vi "scale kalman input.vi"(6 "t scale factor":dbl=2.5e-08, 7 "x scale factors":dbl[](array[numeric])=[0.016, 0.016, 0.00025], 10 "kalman result":T2) -> (2 "kalman result scaled":T1)   [LabVIEW 2010]
uses:
  kalman_result_unscaled.ctl
  kalman_result_scaled.ctl
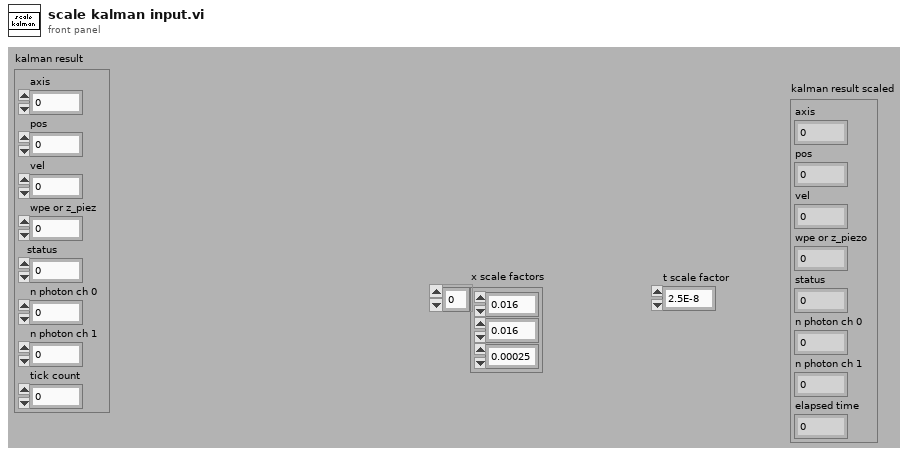
[diagram p1: front panel]
types:
  T1 = typedef "kalman_result_scaled.ctl" = cluster{"axis":u8, "pos":dbl, "vel":dbl, "wpe or z_piezo":dbl, "status":u32, "n photon ch 0":u32, "n photon ch 1":u32, "elapsed time":dbl}
  T2 = typedef "kalman_result_unscaled.ctl" = cluster{"axis":u8, "pos":i16, "vel":i16, "wpe or z_piez":i32, "status":u32, "n photon ch 0":u32, "n photon ch 1":u32, "tick count":u32}
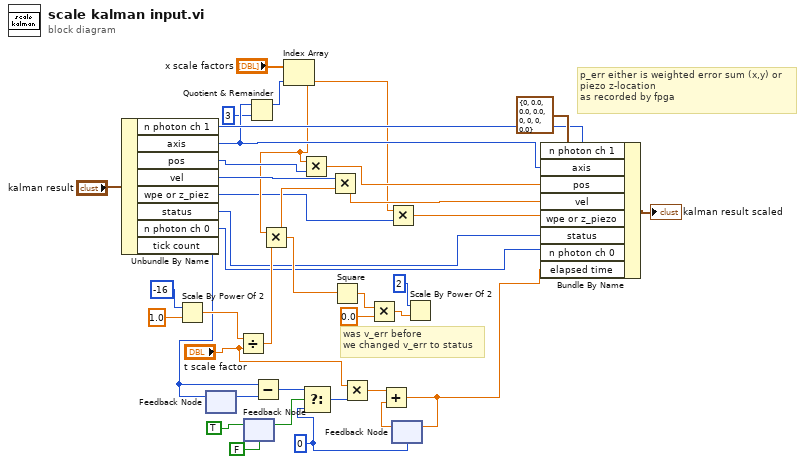
[diagram p0: block diagram]
diagram:
  w16 = 0
  # "was v_err before \nwe changed v_err to status"
  # "p_err either is weighted error sum (x,y) or\npiezo z-location \nas recorded by fpga"
  n1 = Unbundle By Name("kalman result") -> ("n photon ch 1"=w9:u32, "axis"=w6:u8, "pos"=w36:i16, "vel"=w35:i16, "wpe or z_piez"=w2:i32, "status"=w7:u32, "n photon ch 0"=w12:u32, "tick count"=w25:u32)
  n2 = Scale By Power Of 2(n=-16, x=1.0) -> (x*2^n=w32:dbl)
  n3 = feedback-in #1(w25) -> ()
  n4 = feedback #1() -> (w26:u32)  [unwired: 1 in]
  n5 = Divide(x=w32, y="t scale factor") -> (x/y=w31:dbl)
  n6 = feedback-in #2(TRUE ("s")) -> ()
  n7 = feedback #2(FALSE ("s")) -> (w21:bool)
  n8 = Quotient & Remainder(x=w6, y=u8 3) -> (x-y*floor(x/y)=w4:u8)  [unwired: 1 out]
  n9 = Subtract(x=w25, y=w26) -> (x-y=w24:u32)
  n10 = Index Array(array="x scale factors", index=w4) -> (element=w3:dbl)
  n11 = Multiply(x=w3, y=w31) -> (x*y=w30:dbl)
  n12 = Multiply(x=w3, y=w36) -> (x*y=w14:dbl)
  n13 = Select(t=w24, s=w21, f=w16) -> (s? t:f=w20:u32)
  n14 = Multiply(x=w35, y=w30) -> (x*y=w13:dbl)
  n15 = Square(x=w30) -> (x^2=w27:dbl)
  n16 = Multiply(x="t scale factor", y=w20) -> (x*y=w18:dbl)
  n17 = Multiply(x=w27, y=0.0) -> (x*y=w29:dbl)
  n18 = Multiply(x=w3, y=w2) -> (x*y=w1:dbl)
  n19 = feedback #3(w16) -> (w17:dbl)
  n20 = Add(x=w18, y=w17) -> (x+y=w11:dbl)
  n21 = feedback-in #3(w11) -> ()
  n22 = Scale By Power Of 2(n=2, x=w29) -> ()  [unwired: 1 out]
  n23 = Bundle By Name(cluster=T1 {"axis"=0, "pos"=0.0, "vel"=0.0, "wpe or z_piezo"=0.0, "status"=0, "n photon ch 0"=0, "n photon ch 1"=0, "elapsed time"=0.0} ("kalman result scaled"), "n photon ch 1"=w9, "axis"=w6, "pos"=w14, "vel"=w13, "wpe or z_piezo"=w1, "status"=w7, "n photon ch 0"=w12, "elapsed time"=w11) -> (→"kalman result scaled":T1)
